vi "Execute.vi"(8 "error in":errorcluster, 11 "Wait Step in":refnum<class "Wait Step.lvclass">) -> (0 "error out":errorcluster, 1 "Next Step?":bool, 2 "MSG":string, 3 "Wait Step out":refnum<class "Wait Step.lvclass">)   [LabVIEW 2017, in "Controller.lvlib" / "Wait Step.lvclass"]
uses:
  Wait Step.lvclass
  C:/Program Files (x86)/National Instruments/LabVIEW 2017/vi.lib/MSR Consulting, LLC/General Reuse/Sequence/STEPS/STEP.lvclass
  C:/Program Files (x86)/National Instruments/LabVIEW 2017/vi.lib/MSR Consulting, LLC/General Reuse/Sequence/STEPS/LEAVES/Double/Switch DBL.lvclass
  <vilib>/MSR Consulting, LLC/General Reuse/Sequence/STEPS/STEP.lvclass/STEP.ctl
  <vilib>/MSR Consulting, LLC/General Reuse/Sequence/STEPS/LEAVES/Double/Switch DBL.lvclass/Switch DBL.ctl
  <vilib>/MSR Consulting, LLC/General Reuse/Sequence/STEPS/Write First Call.vi
  <vilib>/MSR Consulting, LLC/General Reuse/Sequence/STEPS/Read First Call.vi
  <vilib>/MSR Consulting, LLC/General Reuse/Sequence/STEPS/LEAVES/Double/Read val.vi
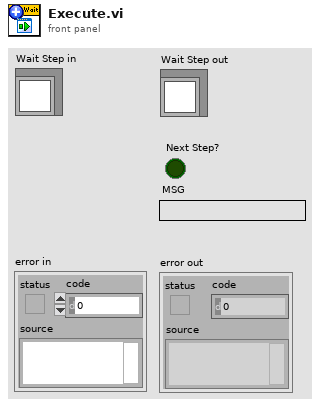
[diagram p1: front panel]
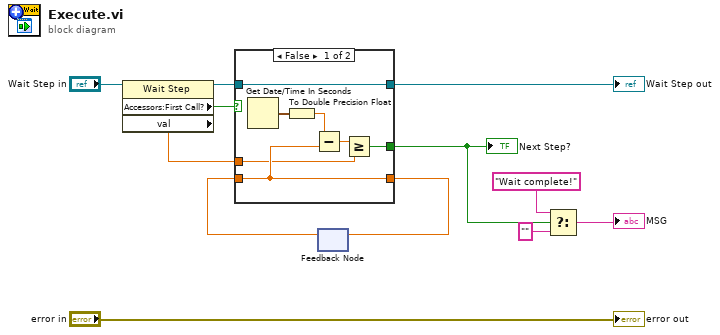
[diagram p0: block diagram]
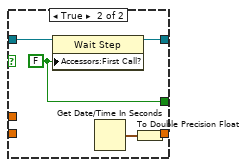
[diagram p2: hidden frame]
diagram:
  n1 = property class="Wait Step"(reference="Wait Step in") -> (reference out=w9:refnum<class "Wait Step.lvclass">, "Accessors:First Call?"=w10:bool, "val"=w5:dbl)  [unwired: 1 in, 1 out]
  n2 = feedback #1() -> (w7:dbl)  [unwired: 1 in]
  n3 = case shown="False" w10 {
    tunnel: w9 -> [w19 w24]
    tunnel: [w13 w23] -> w4
    tunnel: [w16 w21] -> w8
    tunnel: w7 -> [w16 _]
    tunnel: [w19 w22] -> w6
    tunnel: w5 -> [w14 _]
    frame False {
      n4 = Get Date/Time In Seconds() -> (seconds since 1Jan1904=w18:timestamp)
      n5 = To Double Precision Float(number=w18) -> (double precision float=w17:dbl)
      n6 = Subtract(x=w17, y=w16) -> (x-y=w15:dbl)
      n7 = Greater Or Equal?(x=w15, y=w14) -> (x >= y?=w13:bool)
    }
    frame True {
      w23 = FALSE ("First Call?")
      n8 = property class="Wait Step"(reference=w24, "Accessors:First Call?"=w23) -> (reference out=w22:refnum<class "Wait Step.lvclass">)  [unwired: 1 in, 1 out]
      n9 = Get Date/Time In Seconds() -> (seconds since 1Jan1904=w20:timestamp)
      n10 = To Double Precision Float(number=w20) -> (double precision float=w21:dbl)
    }
  }
  "Wait Step out" <- w6
  "Next Step?" <- w4
  n11 = feedback-in #1(w8) -> ()
  n12 = Select(t="Wait complete!" ("MSG"), s=w4, f="") -> (s? t:f=→"MSG":string)
  "error out" <- "error in"
